vi "niRFUtil ERR Check Valid Input (DBL).vi"(0 "Property Value":dbl format="%_3p", 1 "Property Name":string, 7 "Upper Limit":dbl=inf, 9 "Lower Limit":dbl=-inf, 11 "error in (no error)":errorcluster, 12 "Error Code":i32=-379001) -> (15 "error out":errorcluster)   [LabVIEW 2015, in "niRFUtil.lvlib"]
uses:
  niRFUtil.lvlib
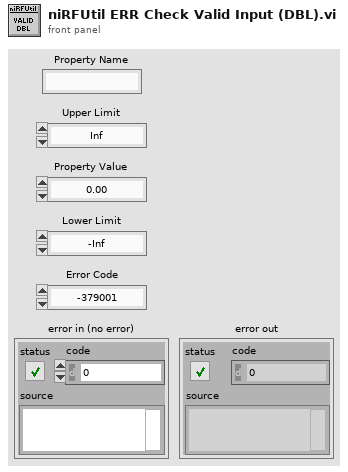
[diagram p1: front panel]
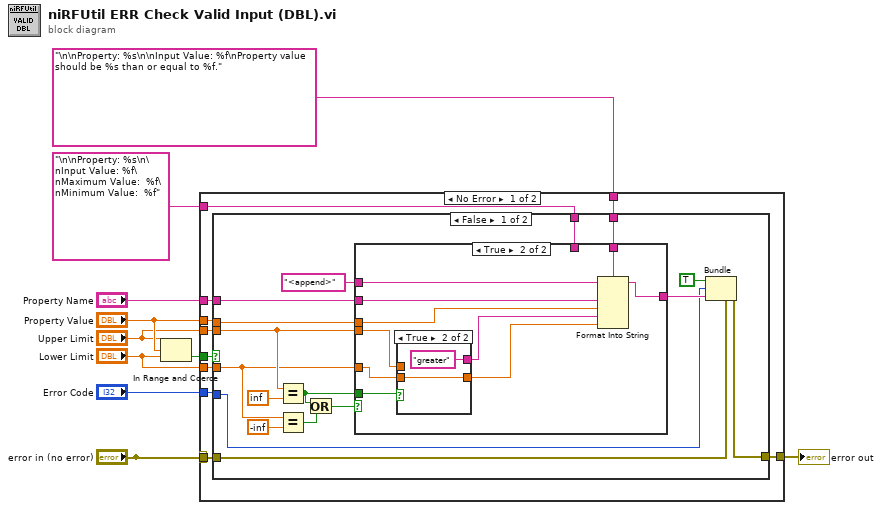
[diagram p0: block diagram]
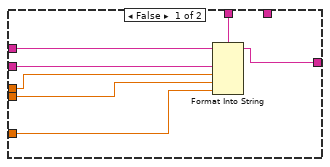
[diagram p2: hidden frame]
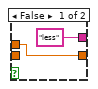
[diagram p3: hidden frame]
diagram:
  n1 = In Range and Coerce(upper limit="Upper Limit", x="Property Value", lower limit="Lower Limit") -> (In Range?=w9:bool)  [unwired: 1 out]
  n2 = case shown="No Error" "error in (no error)" {
    tunnel: "\n\nProperty: %s\n\nInput Value: %f\nMaximum Value:  %f\nMinimum Value:  %f" ("initial string") -> [w20 _]
    tunnel: w9 -> [w19 _]
    tunnel: "\n\nProperty: %s\n\nInput Value: %f\nProperty value should be %s than or equal to %f." ("initial string") -> [w18 _]
    tunnel: "Property Name" -> [w17 _]
    tunnel: "Lower Limit" -> [w16 _]
    tunnel: "Error Code" -> [w15 _]
    tunnel: "error in (no error)" -> [w14 w60]
    tunnel: "Property Value" -> [w13 _]
    tunnel: "Upper Limit" -> [w12 _]
    tunnel: [w11 w60] -> w2
    frame No Error {
      n3 = case shown="False" w19 {
        tunnel: w20 -> [w34 _]
        tunnel: w13 -> [w37 _]
        tunnel: w12 -> [w29 _]
        tunnel: w16 -> [w28 _]
        tunnel: w17 -> [w36 _]
        tunnel: w15 -> [w33 _]
        tunnel: w14 -> [w22 w59]
        tunnel: [w21 w59] -> w11
        tunnel: w18 -> [w32 _]
        frame False {
          n4 = Equal?(x=w29, y=inf) -> (x = y?=w25:bool)
          n5 = Equal?(x=w28, y=-inf) -> (x = y?=w26:bool)
          n6 = Or(x=w25, y=w26) -> (x .or. y?=w27:bool)
          n7 = case shown="True" w27 {
            tunnel: w37 -> [w44 w50]
            tunnel: w29 -> [w43 w47]
            tunnel: w28 -> [w42 w48]
            tunnel: w36 -> [w41 w51]
            tunnel: "<append>" ("message") -> [w40 w54]
            tunnel: [w38 w52] -> w35
            tunnel: w34 -> [w39 _]
            tunnel: w32 -> [_ w53]
            tunnel: w25 -> [_ w45]
            frame False {
              n8 = Format Into String(format string=w39, initial string=w40, w41, w44, w43, w42) -> (resulting string=w38:string)  [unwired: 1 in, 1 out]
            }
            frame True {
              n9 = case shown="True" w45 {
                tunnel: ["less" ("initial string") "greater" ("initial string")] -> w49
                tunnel: w48 -> [_ w57]
                tunnel: w47 -> [w55 _]
                tunnel: [w55 w57] -> w46
                frame False {
                }
                frame True {
                }
              }
              n10 = Format Into String(format string=w53, initial string=w54, w51, w50, w49, w46) -> (resulting string=w52:string)  [unwired: 1 in, 1 out]
            }
          }
          n11 = Bundle(cluster=w22, "status"=TRUE, "code"=w33, "source"=w35) -> (w21:errorcluster)
        }
        frame True {
        }
      }
    }
    frame Error {
    }
  }
  "error out" <- w2
